vi "Output 1-chan.vi"(0 "data":T1[](array[typedef])=[{"I"=0.0, "Q"=0.0, "overflow"=FALSE}, {"I"=0.0, "Q"=0.0, "overflow"=FALSE}], 9 "input valid":bool) -> ()   [LabVIEW 2025]
uses:
  <instrlib>/_niInstr/DSP/v1/Shared/Public/IQ Data.ctl
  <vilib>/rvi/eio/common/nirviEmuTemplateMethod_errors.vi
  <vilib>/eio/EIONode/EIONode.xnode
  <instrlib>/niUSRP/Reference FPGA/Tx Core/niUSRP Tx Core v1 FPGA.lvclass
  C:/Program Files/NI/LVAddons/niidl/1/instr.lib/_niInstr/Instruction Framework/v1/FPGA/Interfaces/Address Space/Address Space.lvclass
  C:/Program Files/NI/LVAddons/niusrprio/1/instr.lib/niUSRP/Reference FPGA/Tx Core/niUSRP Tx Core v1 FPGA.lvclass
  <instrlib>/_niInstr/Basic Elements/v1/FPGA/niInstr Basic Elements v1 FPGA.lvlib
  <instrlib>/_niInstr/DSP/v1/Shared/niInstr DSP v1 Shared.lvlib
  <vilib>/rvi/DataTransferAndStorage/Container/XNode/niFpgaContainer.xnode
  <instrlib>/_niInstr/DSP/v1/FPGA/niInstr DSP v1 FPGA.lvlib
  <vilib>/rvi/FIFO/Fifo_Resource/niFpgaFifoEmulationRefIn.vi
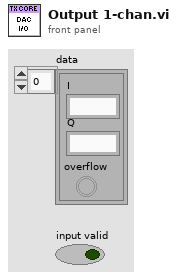
[diagram p1: front panel]
types:
  T1 = typedef "niInstr DSP v1 Shared.lvlib/IQ Data.ctl" = cluster{"I":fxp<+/-,18,1>, "Q":fxp<+/-,18,1>, "overflow":bool}
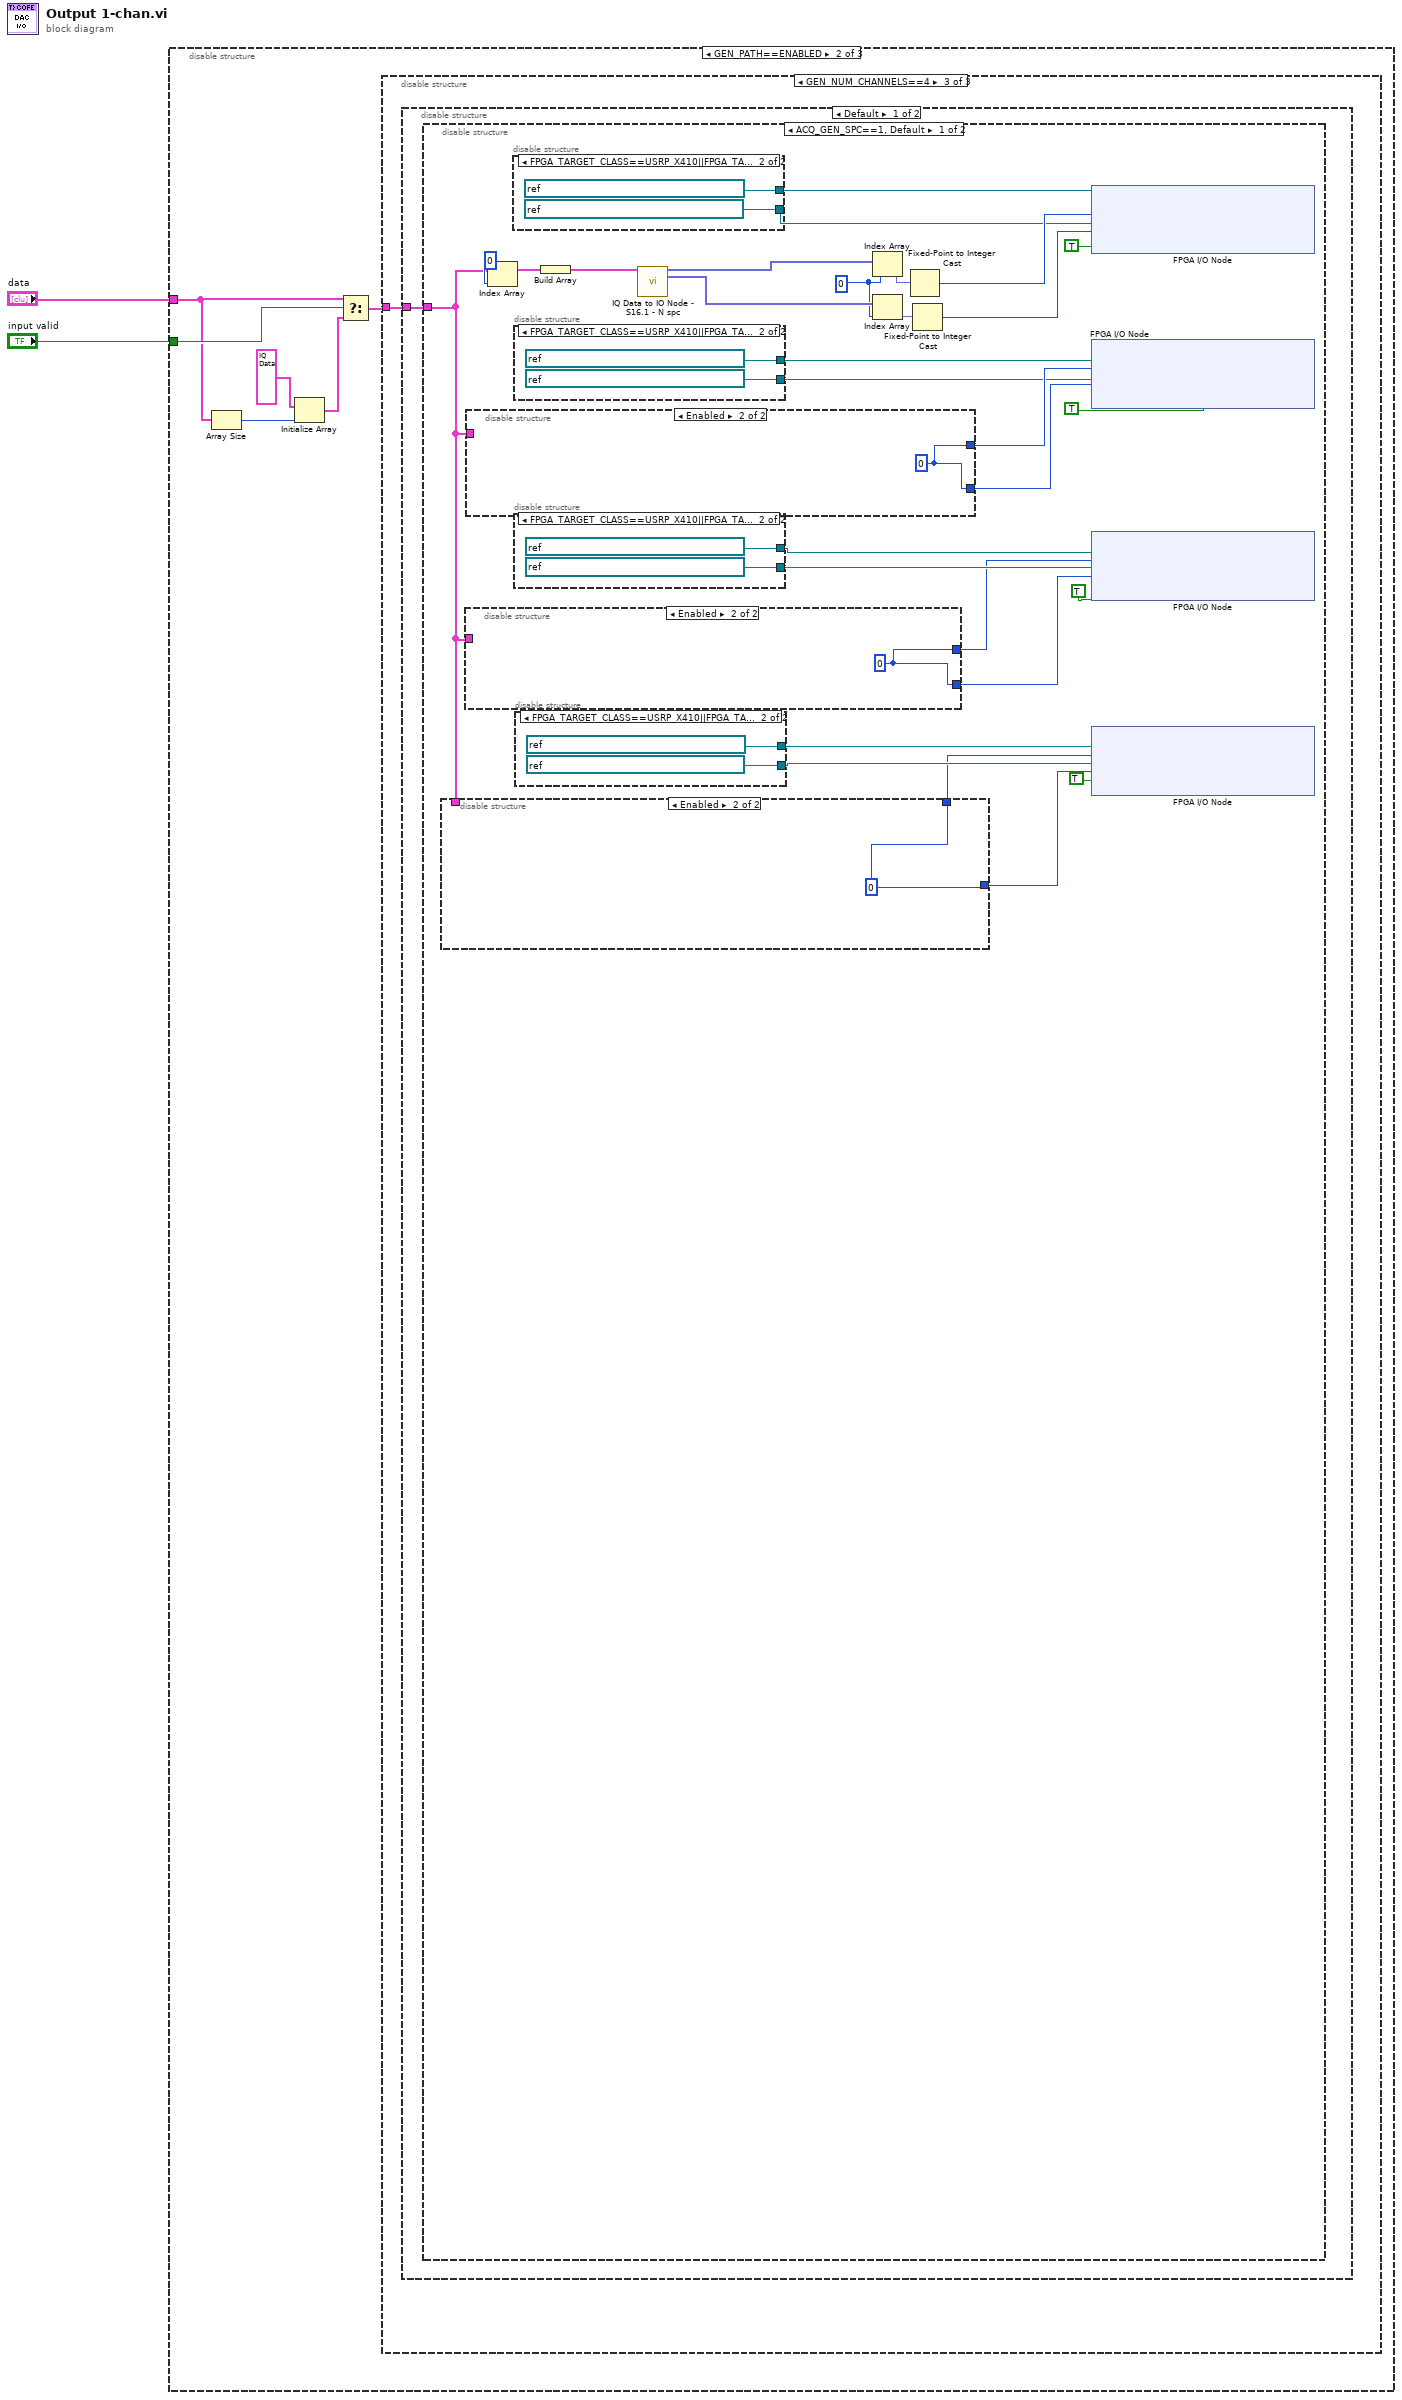
[diagram p0: block diagram]
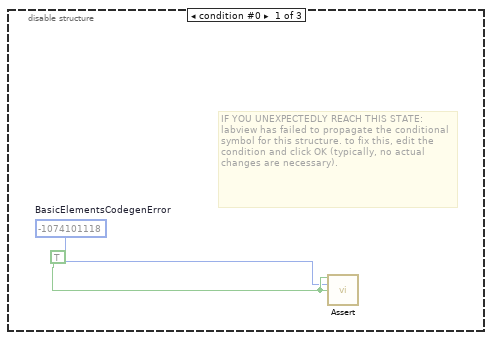
[diagram p2: hidden frame]
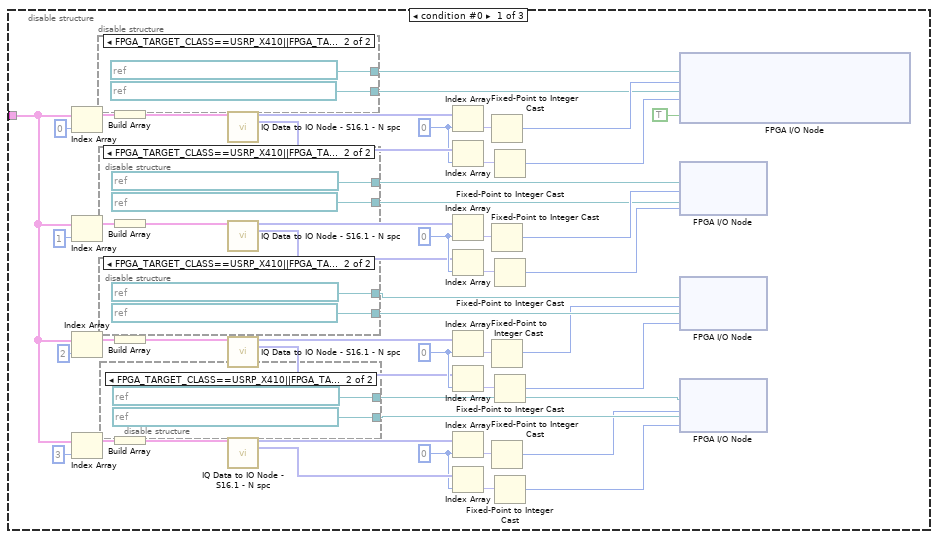
[diagram p4: hidden frame]
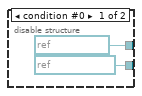
[diagram p5: hidden frame]
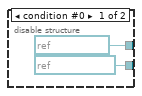
[diagram p6: hidden frame]
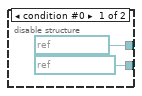
[diagram p7: hidden frame]
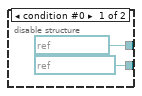
[diagram p8: hidden frame]
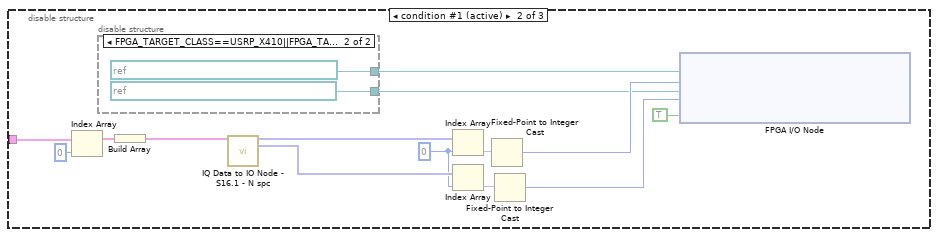
[diagram p9: hidden frame]
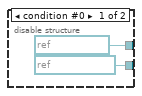
[diagram p10: hidden frame]
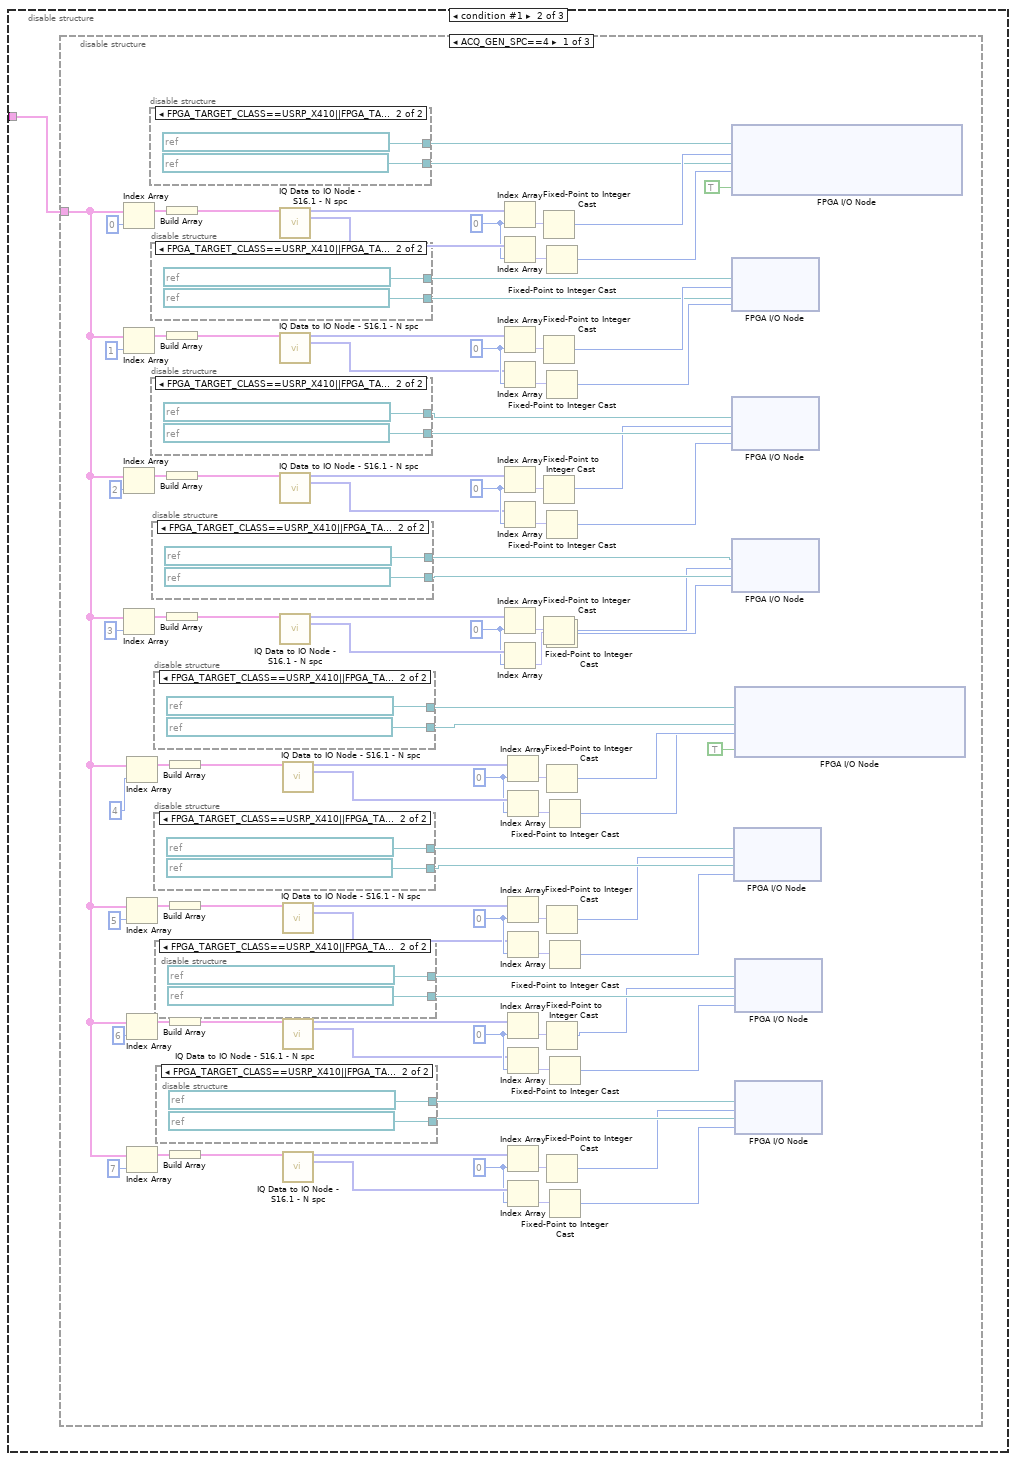
[diagram p11: hidden frame]
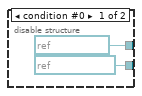
[diagram p12: hidden frame]
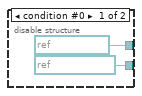
[diagram p13: hidden frame]
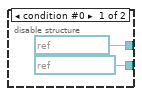
[diagram p14: hidden frame]
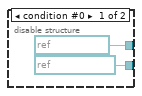
[diagram p15: hidden frame]
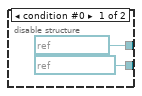
[diagram p16: hidden frame]
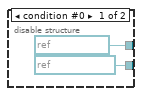
[diagram p17: hidden frame]
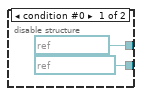
[diagram p18: hidden frame]
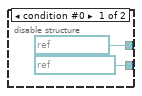
[diagram p19: hidden frame]
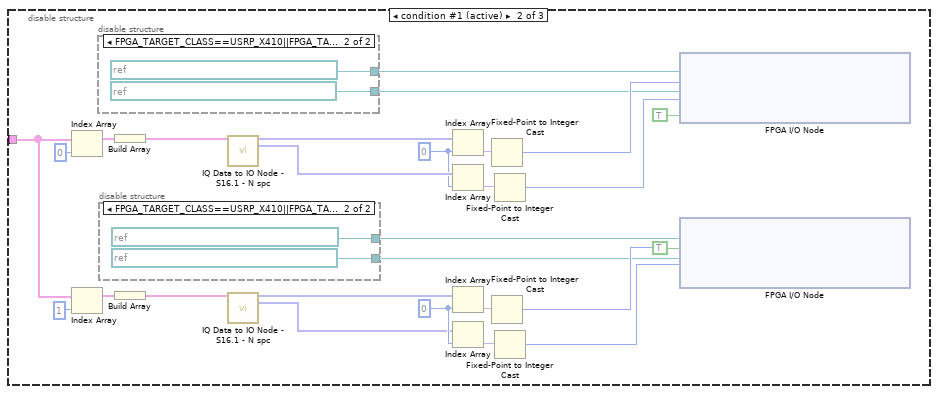
[diagram p20: hidden frame]
diagram:
  n1 = disable-structure shown="GEN_PATH==ENABLED" {
    disable-tunnel: "data" -> [_ w8 _]
    disable-tunnel: "input valid" -> [_ w10 _]
    frame condition #0 {
      w4 = TRUE ("assert")
      w3 = -1074101118  # BasicElementsCodegenError
      # "IF YOU UNEXPECTEDLY REACH THIS STATE:\nlabview has failed to propagate the conditional symbol for this structure. to fix this, edit the condition and click OK (typically, no actual changes are necessary)."
      n2 = call <instrlib>:"Assert.vi"("assert"=w4, "error code"=w3, "enable show error"=w4) -> ()  [unwired: 13 in]
    }
    frame condition #1 (active) {
      n3 = Array Size(array=w8) -> (size(s)=w6:i32)
      n4 = Initialize Array(T1 {"I"=0.0, "Q"=0.0, "overflow"=FALSE} ("data"), w6) -> (w5:T1[])
      n5 = Select(t=w8, s=w10, f=w5) -> (s? t:f=w9:T1[])
      n6 = disable-structure shown="GEN_NUM_CHANNELS==4" {
        disable-tunnel: w9 -> [w11 w96 w263]
        frame condition #0 {
          n7 = disable-structure shown="Default" {
            disable-tunnel: w11 -> [w12 w78 _]
            frame condition #0 {
              w37 = 0 ("index")
              w28 = 0 ("index")
              w47 = 0 ("index")
              w56 = 0 ("index")
              n8 = Index Array(array=w12, index=0) -> (element=w53:T1)
              n9 = Index Array(array=w12, index=1) -> (element=w48:T1)
              n10 = Index Array(array=w12, index=2) -> (element=w30:T1)
              n11 = Index Array(array=w12, index=3) -> (element=w35:T1)
              n12 = disable-structure shown="FPGA_TARGET_CLASS==USRP_X410||FPGA_TARGET_CLASS==USRP_X410__EMBEDDED____UNSUPPORTED" {
                disable-tunnel: [refnum<k21> "RF 0/Tx/I" ("tx regs.i out resource") refnum<k21> "Daughterboard 0\\RF 0.Tx.I0" ("FPGA I/O")] -> w23
                disable-tunnel: [refnum<k21> "RF 0/Tx/Q" ("tx regs.i out resource") refnum<k21> "Daughterboard 0\\RF 0.Tx.Q0" ("FPGA I/O")] -> w22
                frame condition #0 {
                }
                frame condition #1 (active) {
                }
              }
              n13 = disable-structure shown="FPGA_TARGET_CLASS==USRP_X410||FPGA_TARGET_CLASS==USRP_X410__EMBEDDED____UNSUPPORTED" {
                disable-tunnel: [refnum<k21> "RF 0/Tx/I" ("tx regs.i out resource") refnum<k21> "Daughterboard 0\\RF 0.Tx.I1" ("FPGA I/O")] -> w21
                disable-tunnel: [refnum<k21> "RF 0/Tx/Q" ("tx regs.i out resource") refnum<k21> "Daughterboard 0\\RF 0.Tx.Q1" ("FPGA I/O")] -> w20
                frame condition #0 {
                }
                frame condition #1 (active) {
                }
              }
              n14 = disable-structure shown="FPGA_TARGET_CLASS==USRP_X410||FPGA_TARGET_CLASS==USRP_X410__EMBEDDED____UNSUPPORTED" {
                disable-tunnel: [refnum<k21> "RF 0/Tx/I" ("tx regs.i out resource") refnum<k21> "Daughterboard 0\\RF 0.Tx.I2" ("FPGA I/O")] -> w19
                disable-tunnel: [refnum<k21> "RF 0/Tx/Q" ("tx regs.i out resource") refnum<k21> "Daughterboard 0\\RF 0.Tx.Q2" ("FPGA I/O")] -> w18
                frame condition #0 {
                }
                frame condition #1 (active) {
                }
              }
              n15 = disable-structure shown="FPGA_TARGET_CLASS==USRP_X410||FPGA_TARGET_CLASS==USRP_X410__EMBEDDED____UNSUPPORTED" {
                disable-tunnel: [refnum<k21> "RF 0/Tx/I" ("tx regs.i out resource") refnum<k21> "Daughterboard 0\\RF 0.Tx.I3" ("FPGA I/O")] -> w17
                disable-tunnel: [refnum<k21> "RF 0/Tx/Q" ("tx regs.i out resource") refnum<k21> "Daughterboard 0\\RF 0.Tx.Q3" ("FPGA I/O")] -> w16
                frame condition #0 {
                }
                frame condition #1 (active) {
                }
              }
              n16 = Build Array(w53) -> (w51:T1[])
              n17 = Build Array(w48) -> (w50:T1[])
              n18 = Build Array(w30) -> (w32:T1[])
              n19 = Build Array(w35) -> (w33:T1[])
              n20 = call <instrlib>:"IQ Data to IO Node - S16.1 - N spc.vi"("data in"=w51) -> ("I out"=w61:fxp<+/-,16,1>[], "Q out"=w60:fxp<+/-,16,1>[])  [unwired: 12 in, 1 out]
              n21 = call <instrlib>:"IQ Data to IO Node - S16.1 - N spc.vi"("data in"=w50) -> ("I out"=w42:fxp<+/-,16,1>[], "Q out"=w43:fxp<+/-,16,1>[])  [unwired: 12 in, 1 out]
              n22 = call <instrlib>:"IQ Data to IO Node - S16.1 - N spc.vi"("data in"=w32) -> ("I out"=w24:fxp<+/-,16,1>[], "Q out"=w25:fxp<+/-,16,1>[])  [unwired: 12 in, 1 out]
              n23 = call <instrlib>:"IQ Data to IO Node - S16.1 - N spc.vi"("data in"=w33) -> ("I out"=w41:fxp<+/-,16,1>[], "Q out"=w40:fxp<+/-,16,1>[])  [unwired: 12 in, 1 out]
              n24 = Index Array(array=w61, index=w56) -> (element=w59:fxp<+/-,16,1>)
              n25 = Index Array(array=w60, index=w56) -> (element=w57:fxp<+/-,16,1>)
              n26 = Index Array(array=w42, index=w47) -> (element=w44:fxp<+/-,16,1>)
              n27 = Index Array(array=w43, index=w47) -> (element=w46:fxp<+/-,16,1>)
              n28 = Index Array(array=w24, index=w28) -> (element=w26:fxp<+/-,16,1>)
              n29 = Index Array(array=w25, index=w28) -> (element=w27:fxp<+/-,16,1>)
              n30 = Index Array(array=w41, index=w37) -> (element=w39:fxp<+/-,16,1>)
              n31 = Index Array(array=w40, index=w37) -> (element=w38:fxp<+/-,16,1>)
              n32 = Fixed-Point to Integer Cast(1:w59) -> (0:w58:i16)
              n33 = Fixed-Point to Integer Cast(1:w44) -> (0:w45:i16)
              n34 = Fixed-Point to Integer Cast(1:w26) -> (0:w13:i16)
              n35 = Fixed-Point to Integer Cast(1:w39) -> (0:w15:i16)
              n36 = Fixed-Point to Integer Cast(1:w57) -> (0:w55:i16)
              n37 = Fixed-Point to Integer Cast(1:w46) -> (0:w14:i16)
              n38 = Fixed-Point to Integer Cast(1:w27) -> (0:w29:i16)
              n39 = Fixed-Point to Integer Cast(1:w38) -> (0:w36:i16)
              n40 = xnode "FPGA I/O Node"("I/O Item"=w58, "FPGA I/O In"=w23, "I/O Item"=w55, "FPGA I/O In"=w22, "Daughterboard 0\\RF 0.Tx.Data Valid"=TRUE ("Daughterboard 1\\s1TxDbaCh0DataValid")) -> ()  [unwired: 1 in, 3 out]
              n41 = xnode "FPGA I/O Node"("I/O Item"=w45, "FPGA I/O In"=w21, "I/O Item"=w14, "FPGA I/O In"=w20) -> ()  [unwired: 2 out]
              n42 = xnode "FPGA I/O Node"("I/O Item"=w13, "FPGA I/O In"=w19, "I/O Item"=w29, "FPGA I/O In"=w18) -> ()  [unwired: 2 out]
              n43 = xnode "FPGA I/O Node"("I/O Item"=w15, "FPGA I/O In"=w17, "I/O Item"=w36, "FPGA I/O In"=w16) -> ()  [unwired: 2 out]
            }
            frame condition #1 (active) {
              w86 = 0 ("index")
              n44 = Index Array(array=w78, index=0) -> (element=w83:T1)
              n45 = disable-structure shown="FPGA_TARGET_CLASS==USRP_X410||FPGA_TARGET_CLASS==USRP_X410__EMBEDDED____UNSUPPORTED" {
                disable-tunnel: [refnum<k21> "RF 0/Tx/I" ("tx regs.i out resource") refnum<k21> "Daughterboard 0\\RF 0.Tx.I" ("FPGA I/O")] -> w80
                disable-tunnel: [refnum<k21> "RF 0/Tx/Q" ("tx regs.i out resource") refnum<k21> "Daughterboard 0\\RF 0.Tx.Q" ("FPGA I/O")] -> w79
                frame condition #0 {
                }
                frame condition #1 (active) {
                }
              }
              n46 = Build Array(w83) -> (w81:T1[])
              n47 = call <instrlib>:"IQ Data to IO Node - S16.1 - N spc.vi"("data in"=w81) -> ("I out"=w91:fxp<+/-,16,1>[], "Q out"=w90:fxp<+/-,16,1>[])  [unwired: 12 in, 1 out]
              n48 = Index Array(array=w91, index=w86) -> (element=w89:fxp<+/-,16,1>)
              n49 = Index Array(array=w90, index=w86) -> (element=w87:fxp<+/-,16,1>)
              n50 = Fixed-Point to Integer Cast(1:w89) -> (0:w88:i16)
              n51 = Fixed-Point to Integer Cast(1:w87) -> (0:w85:i16)
              n52 = xnode "FPGA I/O Node"("I/O Item"=w88, "FPGA I/O In"=w80, "I/O Item"=w85, "FPGA I/O In"=w79, "Daughterboard 0\\RF 0.Tx.Data Valid"=TRUE ("Daughterboard 1\\s1TxDbaCh0DataValid")) -> ()  [unwired: 1 in, 3 out]
            }
            frame condition #2 {
            }
          }
        }
        frame condition #1 {
          n53 = disable-structure shown="ACQ_GEN_SPC==4" {
            disable-tunnel: w96 -> [w99 w228 _]
            frame condition #0 {
              w125 = 0 ("index")
              w117 = 0 ("index")
              w133 = 0 ("index")
              w142 = 0 ("index")
              w171 = 0 ("index")
              w162 = 0 ("index")
              w181 = 0 ("index")
              w190 = 0 ("index")
              n54 = Index Array(array=w99, index=0) -> (element=w187:T1)
              n55 = Index Array(array=w99, index=1) -> (element=w182:T1)
              n56 = Index Array(array=w99, index=2) -> (element=w164:T1)
              n57 = Index Array(array=w99, index=3) -> (element=w169:T1)
              n58 = Index Array(array=w99, index=4) -> (element=w140:T1)
              n59 = Index Array(array=w99, index=5) -> (element=w135:T1)
              n60 = Index Array(array=w99, index=6) -> (element=w119:T1)
              n61 = Index Array(array=w99, index=7) -> (element=w124:T1)
              n62 = disable-structure shown="FPGA_TARGET_CLASS==USRP_X410||FPGA_TARGET_CLASS==USRP_X410__EMBEDDED____UNSUPPORTED" {
                disable-tunnel: [refnum<k21> "RF 0/Tx/I" ("tx regs.i out resource") refnum<k21> "Daughterboard 0\\RF 0.Tx.I0" ("FPGA I/O")] -> w157
                disable-tunnel: [refnum<k21> "RF 0/Tx/Q" ("tx regs.i out resource") refnum<k21> "Daughterboard 0\\RF 0.Tx.Q0" ("FPGA I/O")] -> w156
                frame condition #0 {
                }
                frame condition #1 (active) {
                }
              }
              n63 = disable-structure shown="FPGA_TARGET_CLASS==USRP_X410||FPGA_TARGET_CLASS==USRP_X410__EMBEDDED____UNSUPPORTED" {
                disable-tunnel: [refnum<k21> "RF 0/Tx/I" ("tx regs.i out resource") refnum<k21> "Daughterboard 0\\RF 0.Tx.I1" ("FPGA I/O")] -> w155
                disable-tunnel: [refnum<k21> "RF 0/Tx/Q" ("tx regs.i out resource") refnum<k21> "Daughterboard 0\\RF 0.Tx.Q1" ("FPGA I/O")] -> w154
                frame condition #0 {
                }
                frame condition #1 (active) {
                }
              }
              n64 = disable-structure shown="FPGA_TARGET_CLASS==USRP_X410||FPGA_TARGET_CLASS==USRP_X410__EMBEDDED____UNSUPPORTED" {
                disable-tunnel: [refnum<k21> "RF 0/Tx/I" ("tx regs.i out resource") refnum<k21> "Daughterboard 0\\RF 0.Tx.I2" ("FPGA I/O")] -> w153
                disable-tunnel: [refnum<k21> "RF 0/Tx/Q" ("tx regs.i out resource") refnum<k21> "Daughterboard 0\\RF 0.Tx.Q2" ("FPGA I/O")] -> w152
                frame condition #0 {
                }
                frame condition #1 (active) {
                }
              }
              n65 = disable-structure shown="FPGA_TARGET_CLASS==USRP_X410||FPGA_TARGET_CLASS==USRP_X410__EMBEDDED____UNSUPPORTED" {
                disable-tunnel: [refnum<k21> "RF 0/Tx/I" ("tx regs.i out resource") refnum<k21> "Daughterboard 0\\RF 0.Tx.I3" ("FPGA I/O")] -> w151
                disable-tunnel: [refnum<k21> "RF 0/Tx/Q" ("tx regs.i out resource") refnum<k21> "Daughterboard 0\\RF 0.Tx.Q3" ("FPGA I/O")] -> w150
                frame condition #0 {
                }
                frame condition #1 (active) {
                }
              }
              n66 = disable-structure shown="FPGA_TARGET_CLASS==USRP_X410||FPGA_TARGET_CLASS==USRP_X410__EMBEDDED____UNSUPPORTED" {
                disable-tunnel: [refnum<k21> "RF 0/Tx/I" ("tx regs.i out resource") refnum<k21> "Daughterboard 0\\RF 1.Tx.I0" ("FPGA I/O")] -> w112
                disable-tunnel: [refnum<k21> "RF 0/Tx/Q" ("tx regs.i out resource") refnum<k21> "Daughterboard 0\\RF 1.Tx.Q0" ("FPGA I/O")] -> w111
                frame condition #0 {
                }
                frame condition #1 (active) {
                }
              }
              n67 = disable-structure shown="FPGA_TARGET_CLASS==USRP_X410||FPGA_TARGET_CLASS==USRP_X410__EMBEDDED____UNSUPPORTED" {
                disable-tunnel: [refnum<k21> "RF 0/Tx/I" ("tx regs.i out resource") refnum<k21> "Daughterboard 0\\RF 1.Tx.I1" ("FPGA I/O")] -> w110
                disable-tunnel: [refnum<k21> "RF 0/Tx/Q" ("tx regs.i out resource") refnum<k21> "Daughterboard 0\\RF 1.Tx.Q1" ("FPGA I/O")] -> w109
                frame condition #0 {
                }
                frame condition #1 (active) {
                }
              }
              n68 = disable-structure shown="FPGA_TARGET_CLASS==USRP_X410||FPGA_TARGET_CLASS==USRP_X410__EMBEDDED____UNSUPPORTED" {
                disable-tunnel: [refnum<k21> "RF 0/Tx/I" ("tx regs.i out resource") refnum<k21> "Daughterboard 0\\RF 1.Tx.I2" ("FPGA I/O")] -> w108
                disable-tunnel: [refnum<k21> "RF 0/Tx/Q" ("tx regs.i out resource") refnum<k21> "Daughterboard 0\\RF 1.Tx.Q2" ("FPGA I/O")] -> w107
                frame condition #0 {
                }
                frame condition #1 (active) {
                }
              }
              n69 = disable-structure shown="FPGA_TARGET_CLASS==USRP_X410||FPGA_TARGET_CLASS==USRP_X410__EMBEDDED____UNSUPPORTED" {
                disable-tunnel: [refnum<k21> "RF 0/Tx/I" ("tx regs.i out resource") refnum<k21> "Daughterboard 0\\RF 1.Tx.I3" ("FPGA I/O")] -> w106
                disable-tunnel: [refnum<k21> "RF 0/Tx/Q" ("tx regs.i out resource") refnum<k21> "Daughterboard 0\\RF 1.Tx.Q3" ("FPGA I/O")] -> w105
                frame condition #0 {
                }
                frame condition #1 (active) {
                }
              }
              n70 = Build Array(w187) -> (w185:T1[])
              n71 = Build Array(w182) -> (w184:T1[])
              n72 = Build Array(w164) -> (w166:T1[])
              n73 = Build Array(w169) -> (w167:T1[])
              n74 = Build Array(w140) -> (w138:T1[])
              n75 = Build Array(w135) -> (w137:T1[])
              n76 = Build Array(w119) -> (w121:T1[])
              n77 = Build Array(w124) -> (w122:T1[])
              n78 = call <instrlib>:"IQ Data to IO Node - S16.1 - N spc.vi"("data in"=w185) -> ("I out"=w195:fxp<+/-,16,1>[], "Q out"=w194:fxp<+/-,16,1>[])  [unwired: 12 in, 1 out]
              n79 = call <instrlib>:"IQ Data to IO Node - S16.1 - N spc.vi"("data in"=w184) -> ("I out"=w176:fxp<+/-,16,1>[], "Q out"=w177:fxp<+/-,16,1>[])  [unwired: 12 in, 1 out]
              n80 = call <instrlib>:"IQ Data to IO Node - S16.1 - N spc.vi"("data in"=w166) -> ("I out"=w158:fxp<+/-,16,1>[], "Q out"=w159:fxp<+/-,16,1>[])  [unwired: 12 in, 1 out]
              n81 = call <instrlib>:"IQ Data to IO Node - S16.1 - N spc.vi"("data in"=w167) -> ("I out"=w175:fxp<+/-,16,1>[], "Q out"=w174:fxp<+/-,16,1>[])  [unwired: 12 in, 1 out]
              n82 = call <instrlib>:"IQ Data to IO Node - S16.1 - N spc.vi"("data in"=w138) -> ("I out"=w146:fxp<+/-,16,1>[], "Q out"=w145:fxp<+/-,16,1>[])  [unwired: 12 in, 1 out]
              n83 = call <instrlib>:"IQ Data to IO Node - S16.1 - N spc.vi"("data in"=w137) -> ("I out"=w129:fxp<+/-,16,1>[], "Q out"=w130:fxp<+/-,16,1>[])  [unwired: 12 in, 1 out]
              n84 = call <instrlib>:"IQ Data to IO Node - S16.1 - N spc.vi"("data in"=w121) -> ("I out"=w113:fxp<+/-,16,1>[], "Q out"=w114:fxp<+/-,16,1>[])  [unwired: 12 in, 1 out]
              n85 = call <instrlib>:"IQ Data to IO Node - S16.1 - N spc.vi"("data in"=w122) -> ("I out"=w128:fxp<+/-,16,1>[], "Q out"=w127:fxp<+/-,16,1>[])  [unwired: 12 in, 1 out]
              n86 = Index Array(array=w195, index=w190) -> (element=w193:fxp<+/-,16,1>)
              n87 = Index Array(array=w194, index=w190) -> (element=w191:fxp<+/-,16,1>)
              n88 = Index Array(array=w176, index=w181) -> (element=w178:fxp<+/-,16,1>)
              n89 = Index Array(array=w177, index=w181) -> (element=w180:fxp<+/-,16,1>)
              n90 = Index Array(array=w158, index=w162) -> (element=w160:fxp<+/-,16,1>)
              n91 = Index Array(array=w159, index=w162) -> (element=w161:fxp<+/-,16,1>)
              n92 = Index Array(array=w175, index=w171) -> (element=w173:fxp<+/-,16,1>)
              n93 = Index Array(array=w174, index=w171) -> (element=w172:fxp<+/-,16,1>)
              n94 = Index Array(array=w146, index=w142) -> (element=w144:fxp<+/-,16,1>)
              n95 = Index Array(array=w145, index=w142) -> (element=w143:fxp<+/-,16,1>)
              n96 = Index Array(array=w129, index=w133) -> (element=w131:fxp<+/-,16,1>)
              n97 = Index Array(array=w130, index=w133) -> (element=w132:fxp<+/-,16,1>)
              n98 = Index Array(array=w113, index=w117) -> (element=w115:fxp<+/-,16,1>)
              n99 = Index Array(array=w114, index=w117) -> (element=w116:fxp<+/-,16,1>)
              n100 = Index Array(array=w128, index=w125) -> (element=w126:fxp<+/-,16,1>)
              n101 = Index Array(array=w127, index=w125) -> (element=w98:fxp<+/-,16,1>)
              n102 = Fixed-Point to Integer Cast(1:w193) -> (0:w192:i16)
              n103 = Fixed-Point to Integer Cast(1:w178) -> (0:w179:i16)
              n104 = Fixed-Point to Integer Cast(1:w160) -> (0:w147:i16)
              n105 = Fixed-Point to Integer Cast(1:w173) -> (0:w149:i16)
              n106 = Fixed-Point to Integer Cast(1:w191) -> (0:w189:i16)
              n107 = Fixed-Point to Integer Cast(1:w180) -> (0:w148:i16)
              n108 = Fixed-Point to Integer Cast(1:w161) -> (0:w163:i16)
              n109 = Fixed-Point to Integer Cast(1:w172) -> (0:w170:i16)
              n110 = Fixed-Point to Integer Cast(1:w144) -> (0:w103:i16)
              n111 = Fixed-Point to Integer Cast(1:w131) -> (0:w101:i16)
              n112 = Fixed-Point to Integer Cast(1:w115) -> (0:w100:i16)
              n113 = Fixed-Point to Integer Cast(1:w126) -> (0:w104:i16)
              n114 = Fixed-Point to Integer Cast(1:w143) -> (0:w102:i16)
              n115 = Fixed-Point to Integer Cast(1:w132) -> (0:w134:i16)
              n116 = Fixed-Point to Integer Cast(1:w116) -> (0:w118:i16)
              n117 = Fixed-Point to Integer Cast(1:w98) -> (0:w97:i16)
              n118 = xnode "FPGA I/O Node"("I/O Item"=w192, "FPGA I/O In"=w157, "I/O Item"=w189, "FPGA I/O In"=w156, "Daughterboard 0\\RF 0.Tx.Data Valid"=TRUE ("Daughterboard 1\\s1TxDbaCh0DataValid")) -> ()  [unwired: 1 in, 3 out]
              n119 = xnode "FPGA I/O Node"("I/O Item"=w179, "FPGA I/O In"=w155, "I/O Item"=w148, "FPGA I/O In"=w154) -> ()  [unwired: 2 out]
              n120 = xnode "FPGA I/O Node"("I/O Item"=w147, "FPGA I/O In"=w153, "I/O Item"=w163, "FPGA I/O In"=w152) -> ()  [unwired: 2 out]
              n121 = xnode "FPGA I/O Node"("I/O Item"=w149, "FPGA I/O In"=w151, "I/O Item"=w170, "FPGA I/O In"=w150) -> ()  [unwired: 2 out]
              n122 = xnode "FPGA I/O Node"("I/O Item"=w101, "FPGA I/O In"=w110, "I/O Item"=w134, "FPGA I/O In"=w109) -> ()  [unwired: 2 out]
              n123 = xnode "FPGA I/O Node"("I/O Item"=w103, "FPGA I/O In"=w112, "I/O Item"=w102, "FPGA I/O In"=w111, "Daughterboard 0\\RF 1.Tx.Data Valid"=TRUE ("Daughterboard 1\\s1TxDbaCh0DataValid")) -> ()  [unwired: 1 in, 3 out]
              n124 = xnode "FPGA I/O Node"("I/O Item"=w100, "FPGA I/O In"=w108, "I/O Item"=w118, "FPGA I/O In"=w107) -> ()  [unwired: 2 out]
              n125 = xnode "FPGA I/O Node"("I/O Item"=w104, "FPGA I/O In"=w106, "I/O Item"=w97, "FPGA I/O In"=w105) -> ()  [unwired: 2 out]
            }
            frame condition #1 (active) {
              w239 = 0 ("index")
              w249 = 0 ("index")
              n126 = Index Array(array=w228, index=0) -> (element=w246:T1)
              n127 = Index Array(array=w228, index=1) -> (element=w241:T1)
              n128 = disable-structure shown="FPGA_TARGET_CLASS==USRP_X410||FPGA_TARGET_CLASS==USRP_X410__EMBEDDED____UNSUPPORTED" {
                disable-tunnel: [refnum<k21> "RF 0/Tx/I" ("tx regs.i out resource") refnum<k21> "Daughterboard 0\\RF 0.Tx.I" ("FPGA I/O")] -> w233
                disable-tunnel: [refnum<k21> "RF 0/Tx/Q" ("tx regs.i out resource") refnum<k21> "Daughterboard 0\\RF 0.Tx.Q" ("FPGA I/O")] -> w232
                frame condition #0 {
                }
                frame condition #1 (active) {
                }
              }
              n129 = disable-structure shown="FPGA_TARGET_CLASS==USRP_X410||FPGA_TARGET_CLASS==USRP_X410__EMBEDDED____UNSUPPORTED" {
                disable-tunnel: [refnum<k21> "RF 0/Tx/I" ("tx regs.i out resource") refnum<k21> "Daughterboard 0\\RF 1.Tx.I" ("FPGA I/O")] -> w231
                disable-tunnel: [refnum<k21> "RF 0/Tx/Q" ("tx regs.i out resource") refnum<k21> "Daughterboard 0\\RF 1.Tx.Q" ("FPGA I/O")] -> w230
                frame condition #0 {
                }
                frame condition #1 (active) {
                }
              }
              n130 = Build Array(w246) -> (w244:T1[])
              n131 = Build Array(w241) -> (w243:T1[])
              n132 = call <instrlib>:"IQ Data to IO Node - S16.1 - N spc.vi"("data in"=w244) -> ("I out"=w254:fxp<+/-,16,1>[], "Q out"=w253:fxp<+/-,16,1>[])  [unwired: 12 in, 1 out]
              n133 = call <instrlib>:"IQ Data to IO Node - S16.1 - N spc.vi"("data in"=w243) -> ("I out"=w234:fxp<+/-,16,1>[], "Q out"=w235:fxp<+/-,16,1>[])  [unwired: 12 in, 1 out]
              n134 = Index Array(array=w254, index=w249) -> (element=w252:fxp<+/-,16,1>)
              n135 = Index Array(array=w253, index=w249) -> (element=w250:fxp<+/-,16,1>)
              n136 = Index Array(array=w234, index=w239) -> (element=w236:fxp<+/-,16,1>)
              n137 = Index Array(array=w235, index=w239) -> (element=w238:fxp<+/-,16,1>)
              n138 = Fixed-Point to Integer Cast(1:w252) -> (0:w251:i16)
              n139 = Fixed-Point to Integer Cast(1:w236) -> (0:w237:i16)
              n140 = Fixed-Point to Integer Cast(1:w250) -> (0:w248:i16)
              n141 = Fixed-Point to Integer Cast(1:w238) -> (0:w229:i16)
              n142 = xnode "FPGA I/O Node"("I/O Item"=w251, "FPGA I/O In"=w233, "I/O Item"=w248, "FPGA I/O In"=w232, "Daughterboard 0\\RF 0.Tx.Data Valid"=TRUE ("Daughterboard 1\\s1TxDbaCh0DataValid")) -> ()  [unwired: 1 in, 3 out]
              n143 = xnode "FPGA I/O Node"("I/O Item"=w237, "FPGA I/O In"=w231, "I/O Item"=w229, "FPGA I/O In"=w230, "Daughterboard 0\\RF 1.Tx.Data Valid"=TRUE ("Daughterboard 1\\s1TxDbaCh0DataValid")) -> ()  [unwired: 1 in, 3 out]
            }
            frame condition #2 {
            }
          }
        }
        frame condition #2 (active) {
          n144 = disable-structure shown="Default" {
            disable-tunnel: w263 -> [w264 w619]
            frame condition #0 (active) {
              n145 = disable-structure shown="ACQ_GEN_SPC==1, Default" {
                disable-tunnel: w264 -> [w265 w397]
                frame condition #0 (active) {
                  w288 = 0 ("index")
                  n146 = disable-structure shown="Enabled" {
                    disable-tunnel: [w323 w329] -> w280
                    disable-tunnel: [w319 w329] -> w268
                    disable-tunnel: w265 -> [w318 _]
                    frame Disabled {
                      w324 = 0 ("index")
                      n147 = Index Array(array=w318, index=3) -> (element=w322:T1)
                      n148 = Build Array(w322) -> (w320:T1[])
                      n149 = call <instrlib>:"IQ Data to IO Node - S16.1 - N spc.vi"("data in"=w320) -> ("I out"=w328:fxp<+/-,16,1>[], "Q out"=w327:fxp<+/-,16,1>[])  [unwired: 12 in, 1 out]
                      n150 = Index Array(array=w328, index=w324) -> (element=w326:fxp<+/-,16,1>)
                      n151 = Index Array(array=w327, index=w324) -> (element=w325:fxp<+/-,16,1>)
                      n152 = Fixed-Point to Integer Cast(1:w326) -> (0:w319:i16)
                      n153 = Fixed-Point to Integer Cast(1:w325) -> (0:w323:i16)
                    }
                    frame Enabled {
                      w329 = i16 0
                    }
                  }
                  n154 = disable-structure shown="Enabled" {
                    disable-tunnel: [w313 w317] -> w277
                    disable-tunnel: [w307 w317] -> w266
                    disable-tunnel: w265 -> [w306 _]
                    frame Disabled {
                      w312 = 0 ("index")
                      n155 = Index Array(array=w306, index=2) -> (element=w314:T1)
                      n156 = Build Array(w314) -> (w316:T1[])
                      n157 = call <instrlib>:"IQ Data to IO Node - S16.1 - N spc.vi"("data in"=w316) -> ("I out"=w308:fxp<+/-,16,1>[], "Q out"=w309:fxp<+/-,16,1>[])  [unwired: 12 in, 1 out]
                      n158 = Index Array(array=w308, index=w312) -> (element=w310:fxp<+/-,16,1>)
                      n159 = Index Array(array=w309, index=w312) -> (element=w311:fxp<+/-,16,1>)
                      n160 = Fixed-Point to Integer Cast(1:w310) -> (0:w307:i16)
                      n161 = Fixed-Point to Integer Cast(1:w311) -> (0:w313:i16)
                    }
                    frame Enabled {
                      w317 = i16 0
                    }
                  }
                  n162 = disable-structure shown="Enabled" {
                    disable-tunnel: [w299 w305] -> w281
                    disable-tunnel: [w295 w305] -> w267
                    disable-tunnel: w265 -> [w294 _]
                    frame Disabled {
                      w301 = 0 ("index")
                      n163 = Index Array(array=w294, index=1) -> (element=w302:T1)
                      n164 = Build Array(w302) -> (w304:T1[])
                      n165 = call <instrlib>:"IQ Data to IO Node - S16.1 - N spc.vi"("data in"=w304) -> ("I out"=w296:fxp<+/-,16,1>[], "Q out"=w297:fxp<+/-,16,1>[])  [unwired: 12 in, 1 out]
                      n166 = Index Array(array=w296, index=w301) -> (element=w298:fxp<+/-,16,1>)
                      n167 = Index Array(array=w297, index=w301) -> (element=w300:fxp<+/-,16,1>)
                      n168 = Fixed-Point to Integer Cast(1:w298) -> (0:w299:i16)
                      n169 = Fixed-Point to Integer Cast(1:w300) -> (0:w295:i16)
                    }
                    frame Enabled {
                      w305 = i16 0
                    }
                  }
                  n170 = Index Array(array=w265, index=0) -> (element=w285:T1)
                  n171 = disable-structure shown="FPGA_TARGET_CLASS==USRP_X410||FPGA_TARGET_CLASS==USRP_X410__EMBEDDED____UNSUPPORTED" {
                    disable-tunnel: [refnum<k21> "RF 0/Tx/I" ("tx regs.i out resource") refnum<k21> "Daughterboard 0\\RF 0.Tx.I" ("FPGA I/O")] -> w276
                    disable-tunnel: [refnum<k21> "RF 0/Tx/Q" ("tx regs.i out resource") refnum<k21> "Daughterboard 0\\RF 0.Tx.Q" ("FPGA I/O")] -> w275
                    frame condition #0 {
                    }
                    frame condition #1 (active) {
                    }
                  }
                  n172 = disable-structure shown="FPGA_TARGET_CLASS==USRP_X410||FPGA_TARGET_CLASS==USRP_X410__EMBEDDED____UNSUPPORTED" {
                    disable-tunnel: [refnum<k21> "RF 0/Tx/I" ("tx regs.i out resource") refnum<k21> "Daughterboard 0\\RF 1.Tx.I" ("FPGA I/O")] -> w274
                    disable-tunnel: [refnum<k21> "RF 0/Tx/Q" ("tx regs.i out resource") refnum<k21> "Daughterboard 0\\RF 1.Tx.Q" ("FPGA I/O")] -> w273
                    frame condition #0 {
                    }
                    frame condition #1 (active) {
                    }
                  }
                  n173 = disable-structure shown="FPGA_TARGET_CLASS==USRP_X410||FPGA_TARGET_CLASS==USRP_X410__EMBEDDED____UNSUPPORTED" {
                    disable-tunnel: [refnum<k21> "RF 0/Tx/I" ("tx regs.i out resource") refnum<k21> "Daughterboard 1\\RF 0.Tx.I" ("FPGA I/O")] -> w272
                    disable-tunnel: [refnum<k21> "RF 0/Tx/Q" ("tx regs.i out resource") refnum<k21> "Daughterboard 1\\RF 0.Tx.Q" ("FPGA I/O")] -> w271
                    frame condition #0 {
                    }
                    frame condition #1 (active) {
                    }
                  }
                  n174 = disable-structure shown="FPGA_TARGET_CLASS==USRP_X410||FPGA_TARGET_CLASS==USRP_X410__EMBEDDED____UNSUPPORTED" {
                    disable-tunnel: [refnum<k21> "RF 0/Tx/I" ("tx regs.i out resource") refnum<k21> "Daughterboard 1\\RF 1.Tx.I" ("FPGA I/O")] -> w270
                    disable-tunnel: [refnum<k21> "RF 0/Tx/Q" ("tx regs.i out resource") refnum<k21> "Daughterboard 1\\RF 1.Tx.Q" ("FPGA I/O")] -> w269
                    frame condition #0 {
                    }
                    frame condition #1 (active) {
                    }
                  }
                  n175 = Build Array(w285) -> (w283:T1[])
                  n176 = call <instrlib>:"IQ Data to IO Node - S16.1 - N spc.vi"("data in"=w283) -> ("I out"=w293:fxp<+/-,16,1>[], "Q out"=w292:fxp<+/-,16,1>[])  [unwired: 12 in, 1 out]
                  n177 = Index Array(array=w293, index=w288) -> (element=w291:fxp<+/-,16,1>)
                  n178 = Index Array(array=w292, index=w288) -> (element=w289:fxp<+/-,16,1>)
                  n179 = Fixed-Point to Integer Cast(1:w291) -> (0:w290:i16)
                  n180 = Fixed-Point to Integer Cast(1:w289) -> (0:w287:i16)
                  n181 = xnode "FPGA I/O Node"("I/O Item"=w290, "FPGA I/O In"=w276, "I/O Item"=w287, "FPGA I/O In"=w275, "Daughterboard 0\\RF 0.Tx.Data Valid"=TRUE ("Daughterboard 1\\s1TxDbaCh0DataValid")) -> ()  [unwired: 1 in, 3 out]
                  n182 = xnode "FPGA I/O Node"("I/O Item"=w281, "FPGA I/O In"=w274, "I/O Item"=w267, "FPGA I/O In"=w273, "Daughterboard 0\\RF 1.Tx.Data Valid"=TRUE ("Daughterboard 1\\s1TxDbaCh0DataValid")) -> ()  [unwired: 1 in, 3 out]
                  n183 = xnode "FPGA I/O Node"("I/O Item"=w266, "FPGA I/O In"=w272, "I/O Item"=w277, "FPGA I/O In"=w271, "Daughterboard 1\\RF 0.Tx.Data Valid"=TRUE ("Daughterboard 1\\s1TxDbaCh0DataValid")) -> ()  [unwired: 1 in, 3 out]
                  n184 = xnode "FPGA I/O Node"("I/O Item"=w268, "FPGA I/O In"=w270, "I/O Item"=w280, "FPGA I/O In"=w269, "Daughterboard 1\\RF 1.Tx.Data Valid"=TRUE ("Daughterboard 1\\s1TxDbaCh0DataValid")) -> ()  [unwired: 1 in, 3 out]
                }
                frame condition #1 {
                  w409 = 0 ("index")
                  w402 = 0 ("index")
                  w418 = 0 ("index")
                  w427 = 0 ("index")
                  w444 = 0 ("index")
                  w437 = 0 ("index")
                  w454 = 0 ("index")
                  w463 = 0 ("index")
                  w482 = 0 ("index")
                  w473 = 0 ("index")
                  w491 = 0 ("index")
                  w500 = 0 ("index")
                  w518 = 0 ("index")
                  w509 = 0 ("index")
                  w528 = 0 ("index")
                  w537 = 0 ("index")
                  n185 = Index Array(array=w397, index=12) -> (element=w424:T1)
                  n186 = Index Array(array=w397, index=13) -> (element=w419:T1)
                  n187 = Index Array(array=w397, index=14) -> (element=w403:T1)
                  n188 = Index Array(array=w397, index=15) -> (element=w408:T1)
                  n189 = Index Array(array=w397, index=0) -> (element=w534:T1)
                  n190 = Index Array(array=w397, index=1) -> (element=w529:T1)
                  n191 = Index Array(array=w397, index=2) -> (element=w511:T1)
                  n192 = Index Array(array=w397, index=3) -> (element=w516:T1)
                  n193 = Index Array(array=w397, index=4) -> (element=w498:T1)
                  n194 = Index Array(array=w397, index=5) -> (element=w493:T1)
                  n195 = Index Array(array=w397, index=6) -> (element=w475:T1)
                  n196 = Index Array(array=w397, index=7) -> (element=w480:T1)
                  n197 = Index Array(array=w397, index=8) -> (element=w460:T1)
                  n198 = Index Array(array=w397, index=9) -> (element=w455:T1)
                  n199 = Index Array(array=w397, index=10) -> (element=w438:T1)
                  n200 = Index Array(array=w397, index=11) -> (element=w443:T1)
                  n201 = disable-structure shown="FPGA_TARGET_CLASS==USRP_X410||FPGA_TARGET_CLASS==USRP_X410__EMBEDDED____UNSUPPORTED" {
                    disable-tunnel: [refnum<k21> "RF 0/Tx/I" ("tx regs.i out resource") refnum<k21> "Daughterboard 0\\RF 0.Tx.I0" ("FPGA I/O")] -> w396
                    disable-tunnel: [refnum<k21> "RF 0/Tx/Q" ("tx regs.i out resource") refnum<k21> "Daughterboard 0\\RF 0.Tx.Q0" ("FPGA I/O")] -> w395
                    frame condition #0 {
                    }
                    frame condition #1 (active) {
                    }
                  }
                  n202 = disable-structure shown="FPGA_TARGET_CLASS==USRP_X410||FPGA_TARGET_CLASS==USRP_X410__EMBEDDED____UNSUPPORTED" {
                    disable-tunnel: [refnum<k21> "RF 0/Tx/I" ("tx regs.i out resource") refnum<k21> "Daughterboard 0\\RF 0.Tx.I1" ("FPGA I/O")] -> w394
                    disable-tunnel: [refnum<k21> "RF 0/Tx/Q" ("tx regs.i out resource") refnum<k21> "Daughterboard 0\\RF 0.Tx.Q1" ("FPGA I/O")] -> w393
                    frame condition #0 {
                    }
                    frame condition #1 (active) {
                    }
                  }
                  n203 = disable-structure shown="FPGA_TARGET_CLASS==USRP_X410||FPGA_TARGET_CLASS==USRP_X410__EMBEDDED____UNSUPPORTED" {
                    disable-tunnel: [refnum<k21> "RF 0/Tx/I" ("tx regs.i out resource") refnum<k21> "Daughterboard 0\\RF 0.Tx.I2" ("FPGA I/O")] -> w392
                    disable-tunnel: [refnum<k21> "RF 0/Tx/Q" ("tx regs.i out resource") refnum<k21> "Daughterboard 0\\RF 0.Tx.Q2" ("FPGA I/O")] -> w391
                    frame condition #0 {
                    }
                    frame condition #1 (active) {
                    }
                  }
                  n204 = disable-structure shown="FPGA_TARGET_CLASS==USRP_X410||FPGA_TARGET_CLASS==USRP_X410__EMBEDDED____UNSUPPORTED" {
                    disable-tunnel: [refnum<k21> "RF 0/Tx/I" ("tx regs.i out resource") refnum<k21> "Daughterboard 0\\RF 0.Tx.I3" ("FPGA I/O")] -> w390
                    disable-tunnel: [refnum<k21> "RF 0/Tx/Q" ("tx regs.i out resource") refnum<k21> "Daughterboard 0\\RF 0.Tx.Q3" ("FPGA I/O")] -> w389
                    frame condition #0 {
                    }
                    frame condition #1 (active) {
                    }
                  }
                  n205 = disable-structure shown="FPGA_TARGET_CLASS==USRP_X410||FPGA_TARGET_CLASS==USRP_X410__EMBEDDED____UNSUPPORTED" {
                    disable-tunnel: [refnum<k21> "RF 0/Tx/I" ("tx regs.i out resource") refnum<k21> "Daughterboard 0\\RF 1.Tx.I0" ("FPGA I/O")] -> w388
                    disable-tunnel: [refnum<k21> "RF 0/Tx/Q" ("tx regs.i out resource") refnum<k21> "Daughterboard 0\\RF 1.Tx.Q0" ("FPGA I/O")] -> w387
                    frame condition #0 {
                    }
                    frame condition #1 (active) {
                    }
                  }
                  n206 = disable-structure shown="FPGA_TARGET_CLASS==USRP_X410||FPGA_TARGET_CLASS==USRP_X410__EMBEDDED____UNSUPPORTED" {
                    disable-tunnel: [refnum<k21> "RF 0/Tx/I" ("tx regs.i out resource") refnum<k21> "Daughterboard 0\\RF 1.Tx.I1" ("FPGA I/O")] -> w386
                    disable-tunnel: [refnum<k21> "RF 0/Tx/Q" ("tx regs.i out resource") refnum<k21> "Daughterboard 0\\RF 1.Tx.Q1" ("FPGA I/O")] -> w385
                    frame condition #0 {
                    }
                    frame condition #1 (active) {
                    }
                  }
                  n207 = disable-structure shown="FPGA_TARGET_CLASS==USRP_X410||FPGA_TARGET_CLASS==USRP_X410__EMBEDDED____UNSUPPORTED" {
                    disable-tunnel: [refnum<k21> "RF 0/Tx/I" ("tx regs.i out resource") refnum<k21> "Daughterboard 0\\RF 1.Tx.I2" ("FPGA I/O")] -> w384
                    disable-tunnel: [refnum<k21> "RF 0/Tx/Q" ("tx regs.i out resource") refnum<k21> "Daughterboard 0\\RF 1.Tx.Q2" ("FPGA I/O")] -> w383
                    frame condition #0 {
                    }
                    frame condition #1 (active) {
                    }
                  }
                  n208 = disable-structure shown="FPGA_TARGET_CLASS==USRP_X410||FPGA_TARGET_CLASS==USRP_X410__EMBEDDED____UNSUPPORTED" {
                    disable-tunnel: [refnum<k21> "RF 0/Tx/I" ("tx regs.i out resource") refnum<k21> "Daughterboard 1\\RF 0.Tx.I0" ("FPGA I/O")] -> w380
                    disable-tunnel: [refnum<k21> "RF 0/Tx/Q" ("tx regs.i out resource") refnum<k21> "Daughterboard 1\\RF 0.Tx.Q0" ("FPGA I/O")] -> w379
                    frame condition #0 {
                    }
                    frame condition #1 (active) {
                    }
                  }
                  n209 = disable-structure shown="FPGA_TARGET_CLASS==USRP_X410||FPGA_TARGET_CLASS==USRP_X410__EMBEDDED____UNSUPPORTED" {
                    disable-tunnel: [refnum<k21> "RF 0/Tx/I" ("tx regs.i out resource") refnum<k21> "Daughterboard 0\\RF 1.Tx.I3" ("FPGA I/O")] -> w382
                    disable-tunnel: [refnum<k21> "RF 0/Tx/Q" ("tx regs.i out resource") refnum<k21> "Daughterboard 0\\RF 1.Tx.Q3" ("FPGA I/O")] -> w381
                    frame condition #0 {
                    }
                    frame condition #1 (active) {
                    }
                  }
                  n210 = disable-structure shown="FPGA_TARGET_CLASS==USRP_X410||FPGA_TARGET_CLASS==USRP_X410__EMBEDDED____UNSUPPORTED" {
                    disable-tunnel: [refnum<k21> "RF 0/Tx/I" ("tx regs.i out resource") refnum<k21> "Daughterboard 1\\RF 0.Tx.I1" ("FPGA I/O")] -> w378
                    disable-tunnel: [refnum<k21> "RF 0/Tx/Q" ("tx regs.i out resource") refnum<k21> "Daughterboard 1\\RF 0.Tx.Q1" ("FPGA I/O")] -> w377
                    frame condition #0 {
                    }
                    frame condition #1 (active) {
                    }
                  }
                  n211 = disable-structure shown="FPGA_TARGET_CLASS==USRP_X410||FPGA_TARGET_CLASS==USRP_X410__EMBEDDED____UNSUPPORTED" {
                    disable-tunnel: [refnum<k21> "RF 0/Tx/I" ("tx regs.i out resource") refnum<k21> "Daughterboard 1\\RF 0.Tx.I2" ("FPGA I/O")] -> w361
                    disable-tunnel: [refnum<k21> "RF 0/Tx/Q" ("tx regs.i out resource") refnum<k21> "Daughterboard 1\\RF 0.Tx.Q2" ("FPGA I/O")] -> w360
                    frame condition #0 {
                    }
                    frame condition #1 (active) {
                    }
                  }
                  n212 = disable-structure shown="FPGA_TARGET_CLASS==USRP_X410||FPGA_TARGET_CLASS==USRP_X410__EMBEDDED____UNSUPPORTED" {
                    disable-tunnel: [refnum<k21> "RF 0/Tx/I" ("tx regs.i out resource") refnum<k21> "Daughterboard 1\\RF 1.Tx.I0" ("FPGA I/O")] -> w365
                    disable-tunnel: [refnum<k21> "RF 0/Tx/Q" ("tx regs.i out resource") refnum<k21> "Daughterboard 1\\RF 1.Tx.Q0" ("FPGA I/O")] -> w364
                    frame condition #0 {
                    }
                    frame condition #1 (active) {
                    }
                  }
                  n213 = disable-structure shown="FPGA_TARGET_CLASS==USRP_X410||FPGA_TARGET_CLASS==USRP_X410__EMBEDDED____UNSUPPORTED" {
                    disable-tunnel: [refnum<k21> "RF 0/Tx/Q" ("tx regs.i out resource") refnum<k21> "Daughterboard 1\\RF 0.Tx.Q3" ("FPGA I/O")] -> w358
                    disable-tunnel: [refnum<k21> "RF 0/Tx/I" ("tx regs.i out resource") refnum<k21> "Daughterboard 1\\RF 0.Tx.I3" ("FPGA I/O")] -> w359
                    frame condition #0 {
                    }
                    frame condition #1 (active) {
                    }
                  }
                  n214 = disable-structure shown="FPGA_TARGET_CLASS==USRP_X410||FPGA_TARGET_CLASS==USRP_X410__EMBEDDED____UNSUPPORTED" {
                    disable-tunnel: [refnum<k21> "RF 0/Tx/I" ("tx regs.i out resource") refnum<k21> "Daughterboard 1\\RF 1.Tx.I1" ("FPGA I/O")] -> w367
                    disable-tunnel: [refnum<k21> "RF 0/Tx/Q" ("tx regs.i out resource") refnum<k21> "Daughterboard 1\\RF 1.Tx.Q1" ("FPGA I/O")] -> w366
                    frame condition #0 {
                    }
                    frame condition #1 (active) {
                    }
                  }
                  n215 = disable-structure shown="FPGA_TARGET_CLASS==USRP_X410||FPGA_TARGET_CLASS==USRP_X410__EMBEDDED____UNSUPPORTED" {
                    disable-tunnel: [refnum<k21> "RF 0/Tx/I" ("tx regs.i out resource") refnum<k21> "Daughterboard 1\\RF 1.Tx.I2" ("FPGA I/O")] -> w371
                    disable-tunnel: [refnum<k21> "RF 0/Tx/Q" ("tx regs.i out resource") refnum<k21> "Daughterboard 1\\RF 1.Tx.Q2" ("FPGA I/O")] -> w370
                    frame condition #0 {
                    }
                    frame condition #1 (active) {
                    }
                  }
                  n216 = disable-structure shown="FPGA_TARGET_CLASS==USRP_X410||FPGA_TARGET_CLASS==USRP_X410__EMBEDDED____UNSUPPORTED" {
                    disable-tunnel: [refnum<k21> "RF 0/Tx/I" ("tx regs.i out resource") refnum<k21> "Daughterboard 1\\RF 1.Tx.I3" ("FPGA I/O")] -> w374
                    disable-tunnel: [refnum<k21> "RF 0/Tx/Q" ("tx regs.i out resource") refnum<k21> "Daughterboard 1\\RF 1.Tx.Q3" ("FPGA I/O")] -> w375
                    frame condition #0 {
                    }
                    frame condition #1 (active) {
                    }
                  }
                  n217 = Build Array(w424) -> (w422:T1[])
                  n218 = Build Array(w419) -> (w421:T1[])
                  n219 = Build Array(w403) -> (w405:T1[])
                  n220 = Build Array(w408) -> (w406:T1[])
                  n221 = Build Array(w534) -> (w532:T1[])
                  n222 = Build Array(w529) -> (w531:T1[])
                  n223 = Build Array(w511) -> (w513:T1[])
                  n224 = Build Array(w516) -> (w514:T1[])
                  n225 = Build Array(w498) -> (w496:T1[])
                  n226 = Build Array(w493) -> (w495:T1[])
                  n227 = Build Array(w475) -> (w477:T1[])
                  n228 = Build Array(w480) -> (w478:T1[])
                  n229 = Build Array(w460) -> (w458:T1[])
                  n230 = Build Array(w455) -> (w457:T1[])
                  n231 = Build Array(w438) -> (w440:T1[])
                  n232 = Build Array(w443) -> (w441:T1[])
                  n233 = call <instrlib>:"IQ Data to IO Node - S16.1 - N spc.vi"("data in"=w422) -> ("I out"=w432:fxp<+/-,16,1>[], "Q out"=w431:fxp<+/-,16,1>[])  [unwired: 12 in, 1 out]
                  n234 = call <instrlib>:"IQ Data to IO Node - S16.1 - N spc.vi"("data in"=w421) -> ("I out"=w414:fxp<+/-,16,1>[], "Q out"=w415:fxp<+/-,16,1>[])  [unwired: 12 in, 1 out]
                  n235 = call <instrlib>:"IQ Data to IO Node - S16.1 - N spc.vi"("data in"=w405) -> ("I out"=w398:fxp<+/-,16,1>[], "Q out"=w399:fxp<+/-,16,1>[])  [unwired: 12 in, 1 out]
                  n236 = call <instrlib>:"IQ Data to IO Node - S16.1 - N spc.vi"("data in"=w406) -> ("I out"=w413:fxp<+/-,16,1>[], "Q out"=w412:fxp<+/-,16,1>[])  [unwired: 12 in, 1 out]
                  n237 = call <instrlib>:"IQ Data to IO Node - S16.1 - N spc.vi"("data in"=w532) -> ("I out"=w542:fxp<+/-,16,1>[], "Q out"=w541:fxp<+/-,16,1>[])  [unwired: 12 in, 1 out]
                  n238 = call <instrlib>:"IQ Data to IO Node - S16.1 - N spc.vi"("data in"=w531) -> ("I out"=w523:fxp<+/-,16,1>[], "Q out"=w524:fxp<+/-,16,1>[])  [unwired: 12 in, 1 out]
                  n239 = call <instrlib>:"IQ Data to IO Node - S16.1 - N spc.vi"("data in"=w513) -> ("I out"=w505:fxp<+/-,16,1>[], "Q out"=w506:fxp<+/-,16,1>[])  [unwired: 12 in, 1 out]
                  n240 = call <instrlib>:"IQ Data to IO Node - S16.1 - N spc.vi"("data in"=w514) -> ("I out"=w522:fxp<+/-,16,1>[], "Q out"=w521:fxp<+/-,16,1>[])  [unwired: 12 in, 1 out]
                  n241 = call <instrlib>:"IQ Data to IO Node - S16.1 - N spc.vi"("data in"=w496) -> ("I out"=w504:fxp<+/-,16,1>[], "Q out"=w503:fxp<+/-,16,1>[])  [unwired: 12 in, 1 out]
                  n242 = call <instrlib>:"IQ Data to IO Node - S16.1 - N spc.vi"("data in"=w495) -> ("I out"=w487:fxp<+/-,16,1>[], "Q out"=w488:fxp<+/-,16,1>[])  [unwired: 12 in, 1 out]
                  n243 = call <instrlib>:"IQ Data to IO Node - S16.1 - N spc.vi"("data in"=w477) -> ("I out"=w469:fxp<+/-,16,1>[], "Q out"=w470:fxp<+/-,16,1>[])  [unwired: 12 in, 1 out]
                  n244 = call <instrlib>:"IQ Data to IO Node - S16.1 - N spc.vi"("data in"=w478) -> ("I out"=w486:fxp<+/-,16,1>[], "Q out"=w485:fxp<+/-,16,1>[])  [unwired: 12 in, 1 out]
                  n245 = call <instrlib>:"IQ Data to IO Node - S16.1 - N spc.vi"("data in"=w458) -> ("I out"=w468:fxp<+/-,16,1>[], "Q out"=w467:fxp<+/-,16,1>[])  [unwired: 12 in, 1 out]
                  n246 = call <instrlib>:"IQ Data to IO Node - S16.1 - N spc.vi"("data in"=w457) -> ("I out"=w449:fxp<+/-,16,1>[], "Q out"=w450:fxp<+/-,16,1>[])  [unwired: 12 in, 1 out]
                  n247 = call <instrlib>:"IQ Data to IO Node - S16.1 - N spc.vi"("data in"=w440) -> ("I out"=w433:fxp<+/-,16,1>[], "Q out"=w434:fxp<+/-,16,1>[])  [unwired: 12 in, 1 out]
                  n248 = call <instrlib>:"IQ Data to IO Node - S16.1 - N spc.vi"("data in"=w441) -> ("I out"=w448:fxp<+/-,16,1>[], "Q out"=w447:fxp<+/-,16,1>[])  [unwired: 12 in, 1 out]
                  n249 = Index Array(array=w432, index=w427) -> (element=w430:fxp<+/-,16,1>)
                  n250 = Index Array(array=w431, index=w427) -> (element=w428:fxp<+/-,16,1>)
                  n251 = Index Array(array=w414, index=w418) -> (element=w416:fxp<+/-,16,1>)
                  n252 = Index Array(array=w415, index=w418) -> (element=w417:fxp<+/-,16,1>)
                  n253 = Index Array(array=w398, index=w402) -> (element=w400:fxp<+/-,16,1>)
                  n254 = Index Array(array=w399, index=w402) -> (element=w401:fxp<+/-,16,1>)
                  n255 = Index Array(array=w413, index=w409) -> (element=w411:fxp<+/-,16,1>)
                  n256 = Index Array(array=w412, index=w409) -> (element=w410:fxp<+/-,16,1>)
                  n257 = Index Array(array=w542, index=w537) -> (element=w540:fxp<+/-,16,1>)
                  n258 = Index Array(array=w541, index=w537) -> (element=w538:fxp<+/-,16,1>)
                  n259 = Index Array(array=w523, index=w528) -> (element=w525:fxp<+/-,16,1>)
                  n260 = Index Array(array=w524, index=w528) -> (element=w527:fxp<+/-,16,1>)
                  n261 = Index Array(array=w505, index=w509) -> (element=w507:fxp<+/-,16,1>)
                  n262 = Index Array(array=w506, index=w509) -> (element=w508:fxp<+/-,16,1>)
                  n263 = Index Array(array=w522, index=w518) -> (element=w520:fxp<+/-,16,1>)
                  n264 = Index Array(array=w521, index=w518) -> (element=w519:fxp<+/-,16,1>)
                  n265 = Index Array(array=w504, index=w500) -> (element=w502:fxp<+/-,16,1>)
                  n266 = Index Array(array=w503, index=w500) -> (element=w501:fxp<+/-,16,1>)
                  n267 = Index Array(array=w487, index=w491) -> (element=w489:fxp<+/-,16,1>)
                  n268 = Index Array(array=w488, index=w491) -> (element=w490:fxp<+/-,16,1>)
                  n269 = Index Array(array=w469, index=w473) -> (element=w471:fxp<+/-,16,1>)
                  n270 = Index Array(array=w470, index=w473) -> (element=w472:fxp<+/-,16,1>)
                  n271 = Index Array(array=w486, index=w482) -> (element=w484:fxp<+/-,16,1>)
                  n272 = Index Array(array=w485, index=w482) -> (element=w483:fxp<+/-,16,1>)
                  n273 = Index Array(array=w468, index=w463) -> (element=w466:fxp<+/-,16,1>)
                  n274 = Index Array(array=w467, index=w463) -> (element=w464:fxp<+/-,16,1>)
                  n275 = Index Array(array=w449, index=w454) -> (element=w451:fxp<+/-,16,1>)
                  n276 = Index Array(array=w450, index=w454) -> (element=w453:fxp<+/-,16,1>)
                  n277 = Index Array(array=w433, index=w437) -> (element=w435:fxp<+/-,16,1>)
                  n278 = Index Array(array=w448, index=w444) -> (element=w446:fxp<+/-,16,1>)
                  n279 = Index Array(array=w447, index=w444) -> (element=w445:fxp<+/-,16,1>)
                  n280 = Index Array(array=w434, index=w437) -> (element=w436:fxp<+/-,16,1>)
                  n281 = Fixed-Point to Integer Cast(1:w540) -> (0:w539:i16)
                  n282 = Fixed-Point to Integer Cast(1:w538) -> (0:w536:i16)
                  n283 = Fixed-Point to Integer Cast(1:w525) -> (0:w526:i16)
                  n284 = Fixed-Point to Integer Cast(1:w527) -> (0:w349:i16)
                  n285 = Fixed-Point to Integer Cast(1:w507) -> (0:w348:i16)
                  n286 = Fixed-Point to Integer Cast(1:w508) -> (0:w510:i16)
                  n287 = Fixed-Point to Integer Cast(1:w520) -> (0:w350:i16)
                  n288 = Fixed-Point to Integer Cast(1:w519) -> (0:w517:i16)
                  n289 = Fixed-Point to Integer Cast(1:w502) -> (0:w352:i16)
                  n290 = Fixed-Point to Integer Cast(1:w501) -> (0:w351:i16)
                  n291 = Fixed-Point to Integer Cast(1:w489) -> (0:w347:i16)
                  n292 = Fixed-Point to Integer Cast(1:w490) -> (0:w492:i16)
                  n293 = Fixed-Point to Integer Cast(1:w471) -> (0:w346:i16)
                  n294 = Fixed-Point to Integer Cast(1:w472) -> (0:w474:i16)
                  n295 = Fixed-Point to Integer Cast(1:w484) -> (0:w353:i16)
                  n296 = Fixed-Point to Integer Cast(1:w483) -> (0:w481:i16)
                  n297 = Fixed-Point to Integer Cast(1:w466) -> (0:w465:i16)
                  n298 = Fixed-Point to Integer Cast(1:w464) -> (0:w462:i16)
                  n299 = Fixed-Point to Integer Cast(1:w451) -> (0:w452:i16)
                  n300 = Fixed-Point to Integer Cast(1:w453) -> (0:w376:i16)
                  n301 = Fixed-Point to Integer Cast(1:w435) -> (0:w354:i16)
                  n302 = Fixed-Point to Integer Cast(1:w436) -> (0:w355:i16)
                  n303 = Fixed-Point to Integer Cast(1:w446) -> (0:w357:i16)
                  n304 = Fixed-Point to Integer Cast(1:w445) -> (0:w356:i16)
                  n305 = Fixed-Point to Integer Cast(1:w430) -> (0:w429:i16)
                  n306 = Fixed-Point to Integer Cast(1:w428) -> (0:w426:i16)
                  n307 = Fixed-Point to Integer Cast(1:w416) -> (0:w363:i16)
                  n308 = Fixed-Point to Integer Cast(1:w417) -> (0:w362:i16)
                  n309 = Fixed-Point to Integer Cast(1:w400) -> (0:w369:i16)
                  n310 = Fixed-Point to Integer Cast(1:w401) -> (0:w368:i16)
                  n311 = Fixed-Point to Integer Cast(1:w411) -> (0:w373:i16)
                  n312 = Fixed-Point to Integer Cast(1:w410) -> (0:w372:i16)
                  n313 = xnode "FPGA I/O Node"("I/O Item"=w429, "FPGA I/O In"=w365, "I/O Item"=w426, "FPGA I/O In"=w364, "Daughterboard 1\\RF 1.Tx.Data Valid"=TRUE ("Daughterboard 1\\s1TxDbaCh0DataValid")) -> ()  [unwired: 1 in, 3 out]
                  n314 = xnode "FPGA I/O Node"("I/O Item"=w363, "FPGA I/O In"=w367, "I/O Item"=w362, "FPGA I/O In"=w366) -> ()  [unwired: 2 out]
                  n315 = xnode "FPGA I/O Node"("I/O Item"=w369, "FPGA I/O In"=w371, "I/O Item"=w368, "FPGA I/O In"=w370) -> ()  [unwired: 2 out]
                  n316 = xnode "FPGA I/O Node"("I/O Item"=w373, "FPGA I/O In"=w374, "I/O Item"=w372, "FPGA I/O In"=w375) -> ()  [unwired: 2 out]
                  n317 = xnode "FPGA I/O Node"("I/O Item"=w539, "FPGA I/O In"=w396, "I/O Item"=w536, "FPGA I/O In"=w395, "Daughterboard 0\\RF 0.Tx.Data Valid"=TRUE ("Daughterboard 1\\s1TxDbaCh0DataValid")) -> ()  [unwired: 1 in, 3 out]
                  n318 = xnode "FPGA I/O Node"("I/O Item"=w526, "FPGA I/O In"=w394, "I/O Item"=w349, "FPGA I/O In"=w393) -> ()  [unwired: 2 out]
                  n319 = xnode "FPGA I/O Node"("I/O Item"=w348, "FPGA I/O In"=w392, "I/O Item"=w510, "FPGA I/O In"=w391) -> ()  [unwired: 2 out]
                  n320 = xnode "FPGA I/O Node"("I/O Item"=w350, "FPGA I/O In"=w390, "I/O Item"=w517, "FPGA I/O In"=w389) -> ()  [unwired: 2 out]
                  n321 = xnode "FPGA I/O Node"("I/O Item"=w352, "FPGA I/O In"=w388, "I/O Item"=w351, "FPGA I/O In"=w387, "Daughterboard 0\\RF 1.Tx.Data Valid"=TRUE ("Daughterboard 1\\s1TxDbaCh0DataValid")) -> ()  [unwired: 1 in, 3 out]
                  n322 = xnode "FPGA I/O Node"("I/O Item"=w347, "FPGA I/O In"=w386, "I/O Item"=w492, "FPGA I/O In"=w385) -> ()  [unwired: 2 out]
                  n323 = xnode "FPGA I/O Node"("I/O Item"=w346, "FPGA I/O In"=w384, "I/O Item"=w474, "FPGA I/O In"=w383) -> ()  [unwired: 2 out]
                  n324 = xnode "FPGA I/O Node"("I/O Item"=w353, "FPGA I/O In"=w382, "I/O Item"=w481, "FPGA I/O In"=w381) -> ()  [unwired: 2 out]
                  n325 = xnode "FPGA I/O Node"("I/O Item"=w465, "FPGA I/O In"=w380, "I/O Item"=w462, "FPGA I/O In"=w379, "Daughterboard 1\\RF 0.Tx.Data Valid"=TRUE ("Daughterboard 1\\s1TxDbaCh0DataValid")) -> ()  [unwired: 1 in, 3 out]
                  n326 = xnode "FPGA I/O Node"("I/O Item"=w452, "FPGA I/O In"=w378, "I/O Item"=w376, "FPGA I/O In"=w377) -> ()  [unwired: 2 out]
                  n327 = xnode "FPGA I/O Node"("I/O Item"=w354, "FPGA I/O In"=w361, "I/O Item"=w355, "FPGA I/O In"=w360) -> ()  [unwired: 2 out]
                  n328 = xnode "FPGA I/O Node"("I/O Item"=w357, "FPGA I/O In"=w359, "I/O Item"=w356, "FPGA I/O In"=w358) -> ()  [unwired: 2 out]
                }
              }
            }
            frame condition #1 {
              n329 = Unbundle By Name() -> (w620:refnum<class "niUSRP Tx Core v1 FPGA.lvclass">, "Loopback FIFO"=w629)
              n330 = Array Size(array=w619) -> (size(s)=w628:i32)
              n331 = Initialize Array(T1 {"I"=0.0, "Q"=0.0, "overflow"=FALSE} ("data"), w628) -> (w626:T1[])
              n332 = feedback #1(w626) -> (w624:T1[])
              n333 = feedback-in #1(w619) -> ()
              n334 = Index Array(array=w624) -> (element #1=w623:T1, element #2=w622:T1, element #3=w618:T1, element #4=w617:T1)  [unwired: 4 in]
              n335 = call <instrlib>:"IQ to U32 - 1 spc - S18.1.vi"("IQ data"=w623) -> ("U32 data"=w621:u32)  [unwired: 13 in, 1 out]
              n336 = call <instrlib>:"IQ to U32 - 1 spc - S18.1.vi"("IQ data"=w622) -> ("U32 data"=w613:u32)  [unwired: 13 in, 1 out]
              n337 = call <instrlib>:"IQ to U32 - 1 spc - S18.1.vi"("IQ data"=w618) -> ("U32 data"=w612:u32)  [unwired: 13 in, 1 out]
              n338 = call <instrlib>:"IQ to U32 - 1 spc - S18.1.vi"("IQ data"=w617) -> ("U32 data"=w611:u32)  [unwired: 13 in, 1 out]
              n339 = To Unsigned Word Integer(number=w621) -> (unsigned 16bit integer=w614:u16)
              n340 = To Unsigned Word Integer(number=w613) -> (unsigned 16bit integer=w610:u16)
              n341 = To Unsigned Word Integer(number=w612) -> (unsigned 16bit integer=w609:u16)
              n342 = To Unsigned Word Integer(number=w611) -> (unsigned 16bit integer=w608:u16)
              n343 = Join Numbers(hi=w614, lo=w610) -> ((hi.lo)=w616:u32)
              n344 = Join Numbers(hi=w609, lo=w608) -> ((hi.lo)=w607:u32)
              n345 = Join Numbers(hi=w616, lo=w607) -> ((hi.lo)=w615:u64)
              n346 = xnode ("FIFO Write")("Element"=w615, "Timeout"=0, "FIFO In"=w629) -> ()  [unwired: 2 out]
            }
          }
        }
      }
    }
    frame condition #2 {
    }
  }
